vi "VCS Is Recorder Running.vi"(8 "error in (no error)":errorcluster, 11 "axis in":cluster{"keyHandle":u32, "nodeId":u16}={"keyHandle"=0, "nodeId"=1}) -> (0 "error out":errorcluster, 1 "isRunning":i32, 3 "axis out":cluster{"keyHandle":u32, "nodeId":u16}={"keyHandle"=0, "nodeId"=1})   [LabVIEW 2017, in "maxonEPOS.lvlib"]
doc: "<B>VCS_IsRecorderRunning</B> returns data recorder status running."
uses:
  Examples/maxonEPOS.lvlib
  Resources/EposCmd.dll
  SSI_Tool/InstrumentsInterfaces/Motordriver/maxon EPOS/Resources/EposCmd64.dll
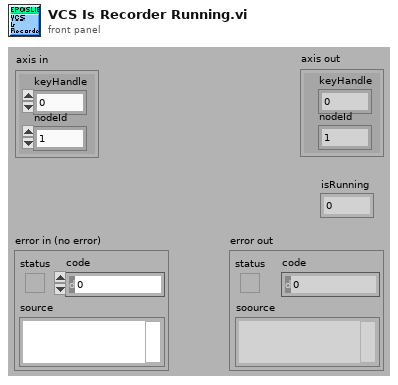
[diagram p1: front panel]
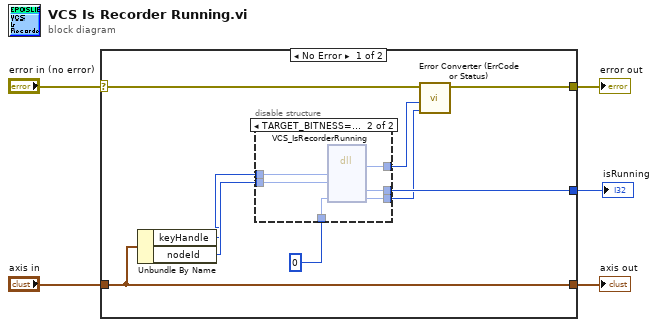
[diagram p0: block diagram]
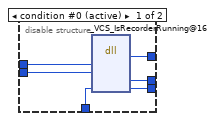
[diagram p2: hidden frame]
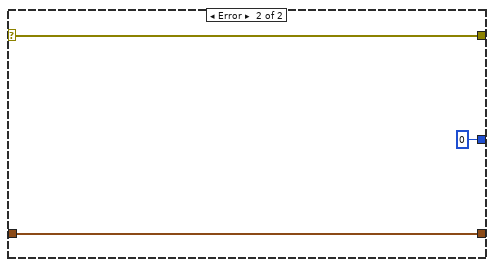
[diagram p3: hidden frame]
diagram:
  n1 = case shown="No Error" "error in (no error)" {
    selector: "error in (no error)" -> [w12 w28]
    tunnel: "axis in" -> [w14 w29]
    tunnel: [w14 w29] -> w4
    tunnel: [w13 w28] -> w3
    tunnel: [w11 0 ("pRunning")] -> w1
    frame No Error {
      n2 = Unbundle By Name(w14) -> ("keyHandle"=w6:u32, "nodeId"=w7:u16)
      n3 = disable-structure shown="TARGET_BITNESS==64" {
        disable-tunnel: [w20 w26] -> w11
        disable-tunnel: [w19 w25] -> w10
        disable-tunnel: [w18 w24] -> w9
        disable-tunnel: u32 0 ("pErrorCode") -> [w17 w23]
        disable-tunnel: w7 -> [w16 w22]
        disable-tunnel: w6 -> [w15 w21]
        frame condition #0 (active) {
          n4 = dll-call lib="C:/workspace/project/scancon/sw/SSI_Tool/InstrumentsInterfaces/Motordriver/maxon EPOS/Resources/EposCmd.*" fn="_VCS_IsRecorderRunning@16"("KeyHandle"=w15, "NodeId"=w16, "pErrorCode"=w17) -> (w19:i32, "pRunning"=w20:i32, "pErrorCode"=w18:u32)  [unwired: 6 in, 2 out]
        }
        frame condition #1 {
          n5 = dll-call lib="C:/Sources/LabView/maxon EPOS/Resources/EposCmd64.*" fn="VCS_IsRecorderRunning" ("EposCmd.dll:_VCS_IsRecorderRunning@16")("KeyHandle"=w21, "NodeId"=w22, "pErrorCode"=w23) -> ("Rückgabetyp"=w25:i32, "pRunning"=w26:i32, "pErrorCode"=w24:u32)  [unwired: 6 in, 2 out]
        }
      }
      n6 = call "Error Converter (ErrCode or Status).vi"("error code"=w9, "return type"=w10, "error in (no error)"=w12) -> ("error out"=w13:errorcluster)  [unwired: 7 in]
    }
    frame Error {
    }
  }
  "isRunning" <- w1
  "error out" <- w3
  "axis out" <- w4
